vi "Get Byte Count.vi"(8 "error in (no error)":errorcluster, 11 "RFFE RegReadExt Command in":refnum<class "RFFE RegReadExt Command.lvclass">) -> (0 "error out":errorcluster, 2 "Byte Count":i32, 3 "RFFE RegReadExt Command out":refnum<class "RFFE RegReadExt Command.lvclass">)   [LabVIEW 2018, in "MIPI RFFE API.lvlib" / "RFFE RegReadExt Command.lvclass"]
uses:
  RFFE RegReadExt Command.lvclass
  RFFE RegReadExt Command.lvclass/RFFE RegReadExt Command.ctl
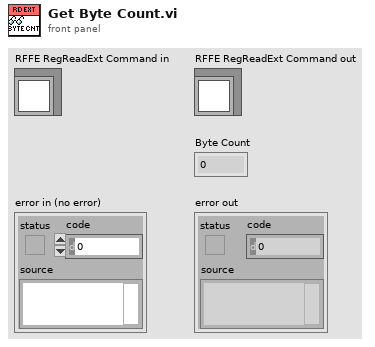
[diagram p1: front panel]
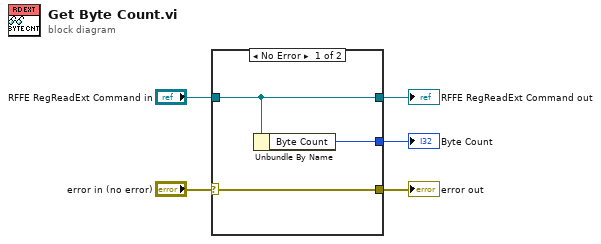
[diagram p0: block diagram]
diagram:
  n1 = case shown="No Error" "error in (no error)" {
    selector: "error in (no error)" -> [w7 w9]
    tunnel: [w8 _] -> w5
    tunnel: "RFFE RegReadExt Command in" -> [w6 w10]
    tunnel: [w7 w9] -> w2
    tunnel: [w6 w10] -> w1
    frame No Error {
      n2 = Unbundle By Name(w6) -> ("Byte Count"=w8:i32)
    }
    frame Error {
    }
  }
  "error out" <- w2
  "RFFE RegReadExt Command out" <- w1
  "Byte Count" <- w5
